vi "readTPDO.vi"(8 "error in (no error)":errorcluster, 10 "TPDO object in":refnum<k20>, 11 "MotorControllerClass in":refnum<class "MotorControllerClass.lvclass">) -> (0 "error out":errorcluster, 1 "TPDO data":u8[](array[numeric]), 2 "TPDO object out":refnum<k20>, 3 "MotorControllerClass out":refnum<class "MotorControllerClass.lvclass">, 5 "new data?":bool)   [LabVIEW 2018, in "MotorControllerClass.lvclass"]
uses:
  BMS/MotorControllerClass.lvclass
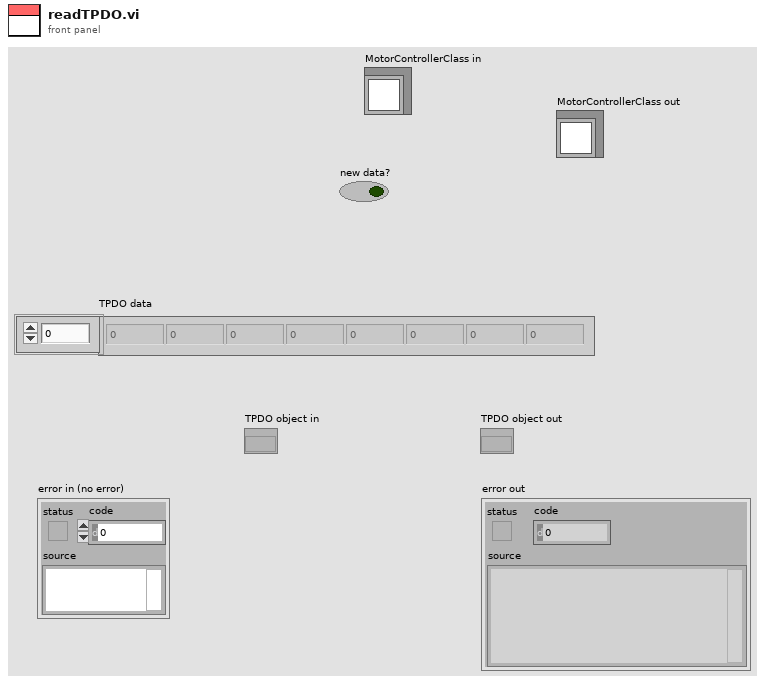
[diagram p1: front panel]
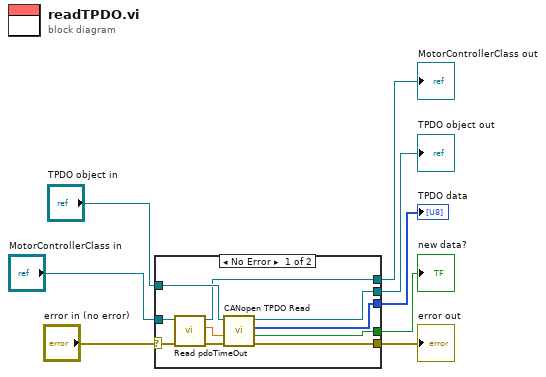
[diagram p0: block diagram]
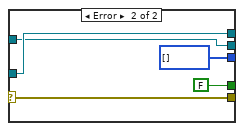
[diagram p2: hidden frame]
diagram:
  n1 = case shown="No Error" "error in (no error)" {
    selector: "error in (no error)" -> [w12 w23]
    tunnel: [w14 w23] -> w7
    tunnel: [w11 w22] -> w1
    tunnel: "MotorControllerClass in" -> [w13 w22]
    tunnel: [w18 u8[] [] ("data")] -> w6
    tunnel: [w17 FALSE ("new data?")] -> w5
    tunnel: "TPDO object in" -> [w16 w19]
    tunnel: [w15 w19] -> w3
    frame No Error {
      n2 = call-dynamic "Read pdoTimeOut.vi"("error in (no error)"=w12, "MotorControllerClass in"=w13) -> ("error out"=w10:errorcluster, "pdoTimeOut"=w9:dbl, "MotorControllerClass out"=w11:refnum<class "MotorControllerClass.lvclass">)  [unwired: 7 in]
      n3 = call <vilib>:"CANopen TPDO Read.vi"("error in (no error)"=w10, "timeout (0s)"=w9, "TPDO object in"=w16) -> ("error out"=w14:errorcluster, "new data?"=w17:bool, "data"=w18:u8[], "TPDO object out"=w15:refnum<k20>)  [unwired: 4 in, 1 out]
    }
    frame Error {
    }
  }
  "MotorControllerClass out" <- w1
  "error out" <- w7
  "TPDO data" <- w6
  "new data?" <- w5
  "TPDO object out" <- w3
